vi "GetChannelList.vi"(8 "error in (no error)":errorcluster, 11 "ByteGSAPIBase in":refnum<class "ByteGSAPIBase.lvclass">) -> (0 "error out":errorcluster, 2 "Channels":cluster{"fields":string[]}, 3 "ByteGSAPIBase out":refnum<class "ByteGSAPIBase.lvclass">)   [LabVIEW 2019, in "ByteGSWebAPI.lvlib" / "ByteGSAPIBase.lvclass"]
uses:
  ByteGSAPIBase.lvclass
  ByteGSAPIBase.lvclass/ByteGSAPIBase.ctl
  <vilib>/Bytelabs/ByteREST/ByteRESTClass/ByteRESTBase/RESTBase.lvclass
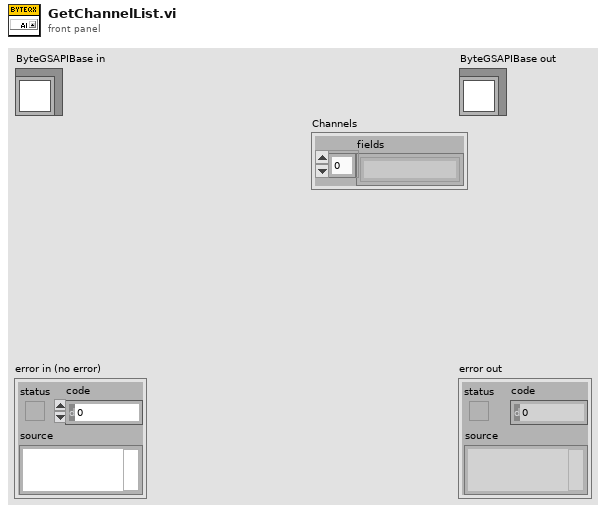
[diagram p1: front panel]
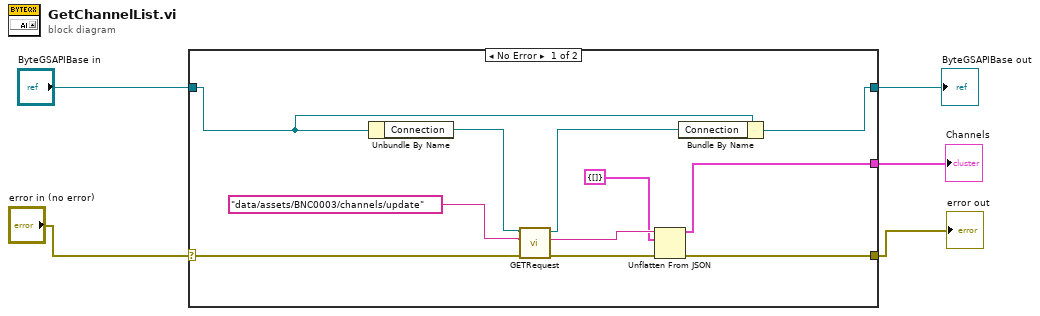
[diagram p0: block diagram]
diagram:
  n1 = case shown="No Error" "error in (no error)" {
    selector: "error in (no error)" -> [w16 w18]
    tunnel: [w8 w18] -> w3
    tunnel: [w14 w17] -> w2
    tunnel: "ByteGSAPIBase in" -> [w15 w17]
    tunnel: [w6 _] -> w1
    frame No Error {
      n2 = Unbundle By Name(w15) -> ("Connection"=w12:refnum<class "RESTBase.lvclass">)
      n3 = call-dynamic "GETRequest.vi"("error in (no error)"=w16, "Request"="data/assets/BNC0003/channels/update", "ByteRESTBase in"=w12) -> ("error out"=w10:errorcluster, "Body"=w9:string, "ByteRESTBase out"=w11:refnum<class "RESTBase.lvclass">)  [unwired: 5 in, 1 out]
      n4 = Unflatten From JSON(JSON string=w9, type and defaults=cluster{"fields":string[]} {"fields"=[]}, error in (no error)=w10) -> (value=w6:cluster{"fields":string[]}, error out=w8:errorcluster)  [unwired: 4 in]
      n5 = Bundle By Name(cluster=w15, "Connection"=w11) -> (w14:refnum<class "ByteGSAPIBase.lvclass">)
    }
    frame Error {
    }
  }
  "error out" <- w3
  "ByteGSAPIBase out" <- w2
  "Channels" <- w1
